vi "Stop Laser.vi"(8 "error in (no error)":errorcluster, 11 "Recipe Process in":refnum<class "Recipe Process.lvclass">) -> (0 "error out":errorcluster, 3 "Recipe Process out":refnum<class "Recipe Process.lvclass">)   [LabVIEW 2022 SP3, in "Recipe Process.lvlib" / "Recipe Process.lvclass"]
uses:
  Recipe Process.lvclass
  Laser/Laser State Data/Laser State.ctl
  Recipe Process.lvclass/Recipe Process.ctl
  Laser/Laser Controller api/Laser API.lvclass
  Laser/Laser State Data/Laser State Data.lvclass
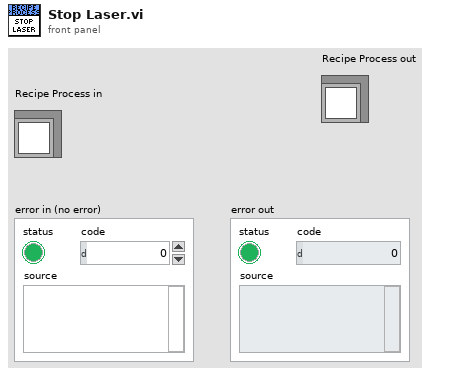
[diagram p1: front panel]
types:
  T1 = typedef "Laser State Data.lvclass/Laser State.ctl" = enum16{"Idle", "Warming", "Ready", "Firing"}
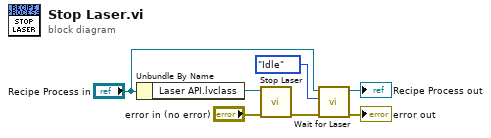
[diagram p0: block diagram]
diagram:
  n1 = Unbundle By Name("Recipe Process in") -> ("Laser API.lvclass"=w7:refnum<class "Laser API.lvclass">)
  n2 = call-dynamic "Stop Laser.vi"("error in (no error)"="error in (no error)", "Laser API in"=w7) -> ("error out"=w3:errorcluster)  [unwired: 8 in, 1 out]
  n3 = call "Wait for Laser.vi"("error in (no error)"=w3, "Desired State"=Laser_State."Idle", "Recipe Process in"="Recipe Process in") -> ("error out"=→"error out":errorcluster, "Recipe Process out"=→"Recipe Process out":refnum<class "Recipe Process.lvclass">)  [unwired: 7 in]
